vi "stopBuildWorkers.vi"(8 "error in (no error)":errorcluster, 11 "BuildServer in":refnum<class "BuildServer.lvclass">) -> (0 "error out":errorcluster, 3 "BuildServer out":refnum<class "BuildServer.lvclass">)   [LabVIEW 2017, in "BuildServer.lvlib" / "BuildServer.lvclass"]
uses:
  BuildServer.lvclass
  Classes/BuildWorker Interface/BuildWorker/BuildWorker.lvclass
  BuildServer.lvclass/BuildServer.ctl
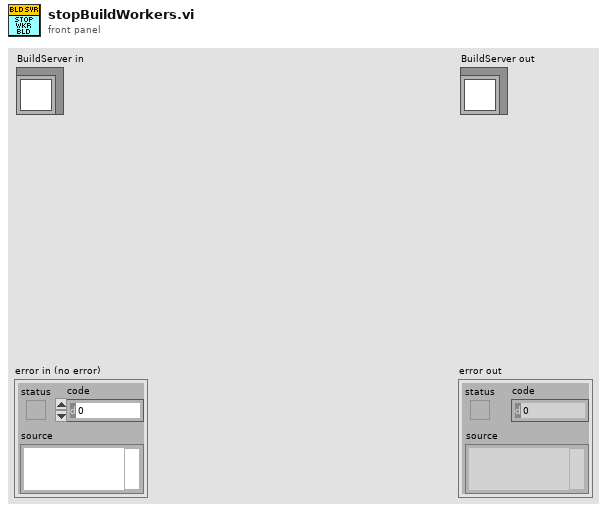
[diagram p1: front panel]
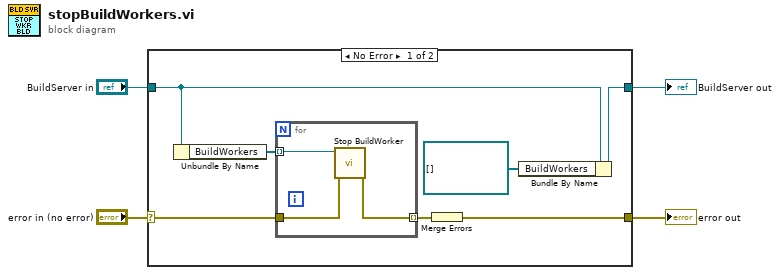
[diagram p0: block diagram]
diagram:
  n1 = case shown="No Error" "error in (no error)" {
    selector: "error in (no error)" -> [w9 w16]
    tunnel: [w7 w16] -> w3
    tunnel: [w6 w15] -> w1
    tunnel: "BuildServer in" -> [w11 w15]
    frame No Error {
      n2 = Unbundle By Name(w11) -> ("BuildWorkers"=w10:refnum<class "BuildWorker.lvclass">[])
      n3 = for {
        tunnel: w10 -> [w14] mode=indexing
        tunnel: w9 -> [w13]
        tunnel: [w12] -> w8 mode=indexing
        n4 = call-dynamic "Stop BuildWorker.vi"("error in (no error)"=w13, "BuildWorker in"=w14) -> ("error out"=w12:errorcluster)  [unwired: 8 in, 1 out]
      }
      n5 = Merge Errors(w8) -> (w7:errorcluster)
      n6 = Bundle By Name(cluster=w11, "BuildWorkers"=refnum<class "BuildWorker.lvclass">[] []) -> (w6:refnum<class "BuildServer.lvclass">)
    }
    frame Error {
    }
  }
  "error out" <- w3
  "BuildServer out" <- w1
